vi "make subs for logging.vi"(11 "spreadsheet string":string) -> (0 "error out":errorcluster, 3 "trimmed string":string)   [LabVIEW 2018]
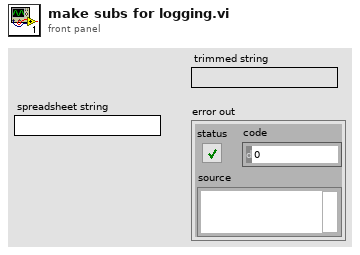
[diagram p1: front panel]
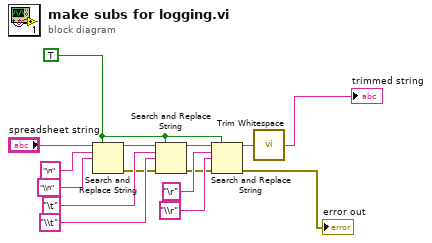
[diagram p0: block diagram]
diagram:
  w14 = TRUE ("want seconds? (F)")
  n1 = Search and Replace String(replace all?=w14, input string="spreadsheet string", search string="\n" ("input string"), replace string="\\n" ("input string")) -> (result string=w4:string, error out=w5:errorcluster)  [unwired: 4 in, 2 out]
  n2 = Search and Replace String(replace all?=w14, input string=w4, search string="\t" ("input string"), replace string="\\t" ("input string"), error in=w5) -> (result string=w10:string, error out=w8:errorcluster)  [unwired: 3 in, 2 out]
  n3 = Search and Replace String(replace all?=w14, input string=w10, search string="\r" ("input string"), replace string="\\r" ("input string"), error in=w8) -> (result string=w9:string, error out=→"error out":errorcluster)  [unwired: 3 in, 2 out]
  n4 = call <vilib>:"Trim Whitespace.vi"("string"=w9) -> ("trimmed string"=→"trimmed string":string)  [unwired: 1 in]
